vi "Parse Package Details.vi"(6 "Repo URL":string, 8 "error in (no error)":errorcluster, 9 "Package Version":string, 10 "Package Name":string, 11 "Repo file in":T1) -> (0 "error out":errorcluster, 2 "Pkg Version":refnum<class "Package Version.lvclass">, 3 "Repo file out":T1)   [LabVIEW 2016, in "Packages.lvlib" / "VIPM.lvlib"]
uses:
  VIPM.lvlib
  Package Version_class/Package Version.lvclass
  <vilib>/Utility/config.llb/Config Data RefNum.ctl
  Package Version_class/Package Version.lvclass/Package Version.ctl
  Package Version_class/Write Name.vi
  Package Version_class/Write Version.vi
  Package Version_class/Write ReleaseDate.vi
  Package Version_class/Write PackageURL.vi
  Package Version_class/Write IconURL.vi
  Package Version_class/Write DisplayName.vi
  Package Version_class/Write Description.vi
  Package Version_class/Write Vendor.vi
  Package Version_class/Write Author.vi
  Package Version_class/Write Release Notes.vi
  Package Version_class/Write Dependencies.vi
  <vilib>/Utility/config.llb/Read Key (String).vi
  <vilib>/Utility/config.llb/NI_LVConfig.lvlib
  <vilib>/httpClient/LabVIEWHTTPClient.lvlib
  WSsupport/WSsupport.lvlib
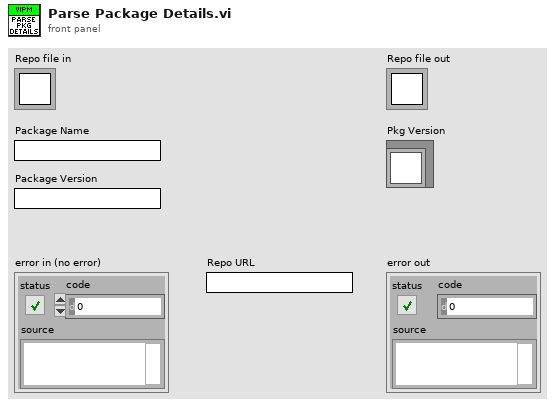
[diagram p1: front panel]
types:
  T1 = typedef "NI_LVConfig.lvlib/Config Data RefNum.ctl" = refnum<k1>
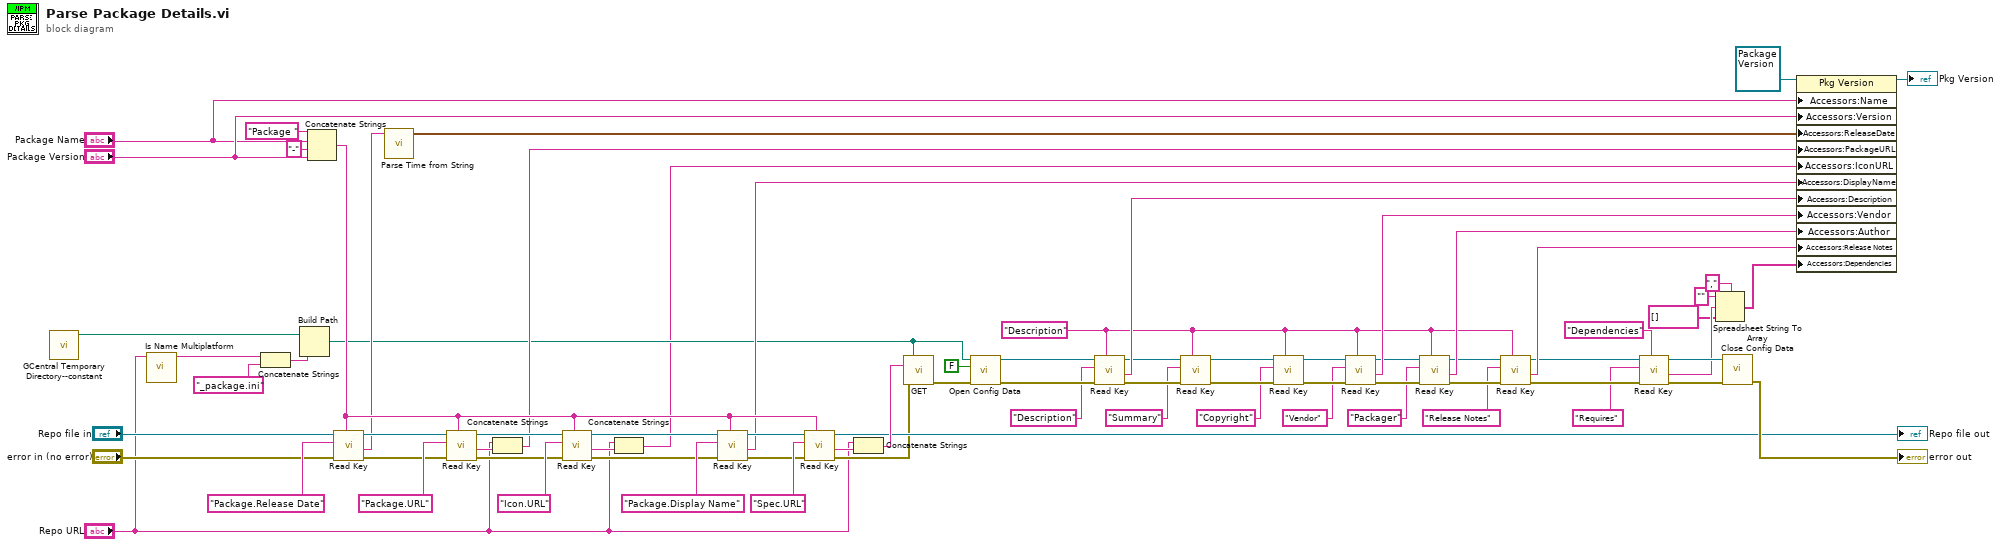
[diagram p0: block diagram]
diagram:
  w55 = "Description" ("section")
  n1 = call "GCentral Temporary Directory--constant.vi"() -> ("GCentral Temporary Directory"=w9:path)  [unwired: 11 in]
  n2 = call <vilib>:"Is Name Multiplatform.vi"("filename"="Repo URL") -> ("suggested filename"=w6:string)  [unwired: 6 in, 4 out]
  n3 = Concatenate Strings(w6, "_package.ini" ("string")) -> (w5:string)
  n4 = Build Path(base path=w9, name or relative path=w5) -> (appended path=w10:path)
  n5 = Concatenate Strings("Package " ("string"), "Package Name", "-" ("string"), "Package Version") -> (w35:string)
  n6 = call-poly <vilib>:"Read Key.vi"("section"=w35, "error in (no error)"="error in (no error)", "key"="Package.Release Date", "refnum"="Repo file in") -> ("error out"=w13:errorcluster, "value"=w16:string, "refnum out"=w20:T1)  [unwired: 4 in, 1 out]
  n7 = call "Parse Time from String.vi"("Time string"=w16) -> ("Timestamp"=w17:timestamp)  [unwired: 10 in]
  n8 = call-poly <vilib>:"Read Key.vi"("section"=w35, "error in (no error)"=w13, "key"="Package.URL", "refnum"=w20) -> ("error out"=w19:errorcluster, "value"=w22:string, "refnum out"=w25:T1)  [unwired: 4 in, 1 out]
  n9 = Concatenate Strings("Repo URL", w22) -> (w23:string)
  n10 = call-poly <vilib>:"Read Key.vi"("section"=w35, "error in (no error)"=w19, "key"="Icon.URL", "refnum"=w25) -> ("error out"=w24:errorcluster, "value"=w27:string, "refnum out"=w29:T1)  [unwired: 4 in, 1 out]
  n11 = Concatenate Strings("Repo URL", w27) -> (w4:string)
  n12 = call-poly <vilib>:"Read Key.vi"("section"=w35, "error in (no error)"=w24, "key"="Package.Display Name", "refnum"=w29) -> ("error out"=w28:errorcluster, "value"=w31:string, "refnum out"=w33:T1)  [unwired: 4 in, 1 out]
  n13 = call-poly <vilib>:"Read Key.vi"("section"=w35, "error in (no error)"=w28, "key"="Spec.URL", "refnum"=w33) -> ("error out"=w32:errorcluster, "value"=w37:string, "refnum out"=→"Repo file out":T1)  [unwired: 4 in, 1 out]
  n14 = Concatenate Strings("Repo URL", w37) -> (w39:string)
  n15 = call <vilib>:"GET.vi"("output file"=w10, "url"=w39, "error in (no error)"=w32) -> ("error out"=w38:errorcluster)  [unwired: 9 in, 3 out]
  n16 = call <vilib>:"Open Config Data.vi"("error in (no error)"=w38, "create file if necessary (T)"=FALSE, "configuration file path"=w10) -> ("error out"=w69:errorcluster, "refnum"=w68:T1)  [unwired: 6 in, 1 out]
  n17 = call-poly <vilib>:"Read Key.vi"("section"=w55, "error in (no error)"=w69, "key"="Description", "refnum"=w68) -> ("error out"=w44:errorcluster, "value"=w71:string, "refnum out"=w43:T1)  [unwired: 4 in, 1 out]
  n18 = call-poly <vilib>:"Read Key.vi"("section"=w55, "error in (no error)"=w44, "key"="Summary", "refnum"=w43) -> ("error out"=w47:errorcluster, "refnum out"=w46:T1)  [unwired: 4 in, 2 out]
  n19 = call-poly <vilib>:"Read Key.vi"("section"=w55, "error in (no error)"=w47, "key"="Copyright", "refnum"=w46) -> ("error out"=w50:errorcluster, "refnum out"=w49:T1)  [unwired: 4 in, 2 out]
  n20 = call-poly <vilib>:"Read Key.vi"("section"=w55, "error in (no error)"=w50, "key"="Vendor", "refnum"=w49) -> ("error out"=w53:errorcluster, "value"=w72:string, "refnum out"=w52:T1)  [unwired: 4 in, 1 out]
  n21 = call-poly <vilib>:"Read Key.vi"("section"=w55, "error in (no error)"=w53, "key"="Packager", "refnum"=w52) -> ("error out"=w57:errorcluster, "value"=w73:string, "refnum out"=w56:T1)  [unwired: 4 in, 1 out]
  n22 = call-poly <vilib>:"Read Key.vi"("section"=w55, "error in (no error)"=w57, "key"="Release Notes", "refnum"=w56) -> ("error out"=w60:errorcluster, "value"=w74:string, "refnum out"=w59:T1)  [unwired: 4 in, 1 out]
  n23 = call-poly <vilib>:"Read Key.vi"("section"="Dependencies", "error in (no error)"=w60, "key"="Requires", "refnum"=w59) -> ("error out"=w67:errorcluster, "value"=w65:string, "refnum out"=w66:T1)  [unwired: 4 in, 1 out]
  n24 = Spreadsheet String To Array(delimiter (Tab)=",", format string="", spreadsheet string=w65, array type (2D Dbl)=string[] []) -> (array=w75:string[])
  n25 = call <vilib>:"Close Config Data.vi"("error in (no error)"=w67, "refnum"=w66) -> ("error out"=→"error out":errorcluster)  [unwired: 8 in, 1 out]
  n26 = property class="Pkg Version"(reference=refnum<class "Package Version.lvclass"> refnum ("Packages.lvlib:Pkg Version"), "Accessors:Name"="Package Name", "Accessors:Version"="Package Version", "Accessors:ReleaseDate"=w17, "Accessors:PackageURL"=w23, "Accessors:IconURL"=w4, "Accessors:DisplayName"=w31, "Accessors:Description"=w71, "Accessors:Vendor"=w72, "Accessors:Author"=w73, "Accessors:Release Notes"=w74, "Accessors:Dependencies"=w75) -> (reference out=→"Pkg Version":refnum<class "Package Version.lvclass">)  [unwired: 1 in, 1 out]
